vi "DFD Integer Delay.vi"   [LabVIEW 2017, in "NI_DigFilterLicensed.lvlib"]
doc: "Delays a signal continuously by a specified integer number of sample intervals. Wire data to the <B>signal in</B> input to determine the polymorphic instance to use or manually select the instance."
uses:
  <vilib>/addons/Digital Filter Design/NI_DigFilterLicensed.lvlib
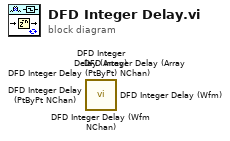
[diagram p0: block diagram]
diagram:
  n1 = call <vilib>:"DFD Integer Delay (Wfm NChan).vi"() -> ()  [unwired: 10 in, 2 out]
  n2 = call <vilib>:"DFD Integer Delay (Array NChan).vi"() -> ()  [unwired: 10 in, 2 out]
  n3 = call <vilib>:"DFD Integer Delay (PtByPt NChan).vi"() -> ()  [unwired: 10 in, 2 out]
  n4 = call <vilib>:"DFD Integer Delay (Wfm).vi"() -> ()  [unwired: 10 in, 2 out]
  n5 = call <vilib>:"DFD Integer Delay (PtByPt).vi"() -> ()  [unwired: 10 in, 2 out]
  n6 = call <vilib>:"DFD Integer Delay (Array).vi"() -> ()  [unwired: 10 in, 2 out]
